vi "Read Attribute Data.vi"(8 "error in (no error)":errorcluster, 10 "Object Name":string, 11 "CS++Factory in":refnum<class "CS++Factory.lvclass">) -> (0 "error out":errorcluster, 2 "Attribute Data":variant, 3 "CS++Factory out":refnum<class "CS++Factory.lvclass">)   [LabVIEW 2013, in "CS++BaseClasses.lvlib" / "CS++Factory.lvclass"]
doc: "Read object attribute data from storage medium.\n\nThe default implementation reads from ini-file."
uses:
  CS++Factory.lvclass
  CS++Factory.lvclass/CS++Factory.ctl
  Libraries/Base/Error Definition.ctl
  <vilib>/Utility/config.llb/Read Key (String).vi
  <vilib>/Utility/config.llb/NI_LVConfig.lvlib
  Libraries/Base/CS++Base.lvlib
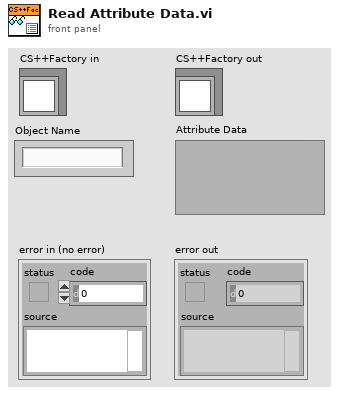
[diagram p1: front panel]
types:
  T1 = typedef "NI_LVConfig.lvlib/Config Data RefNum.ctl" = refnum<k1>
  T2 = typedef "CS++Base.lvlib/Error Definition.ctl" = u16
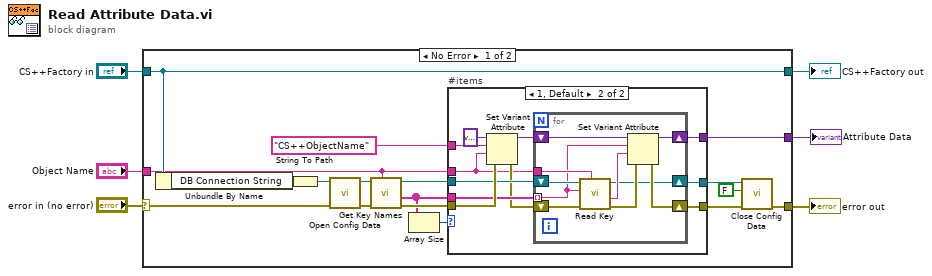
[diagram p0: block diagram]
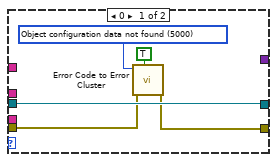
[diagram p2: hidden frame]
diagram:
  n1 = case shown="No Error" "error in (no error)" {
    selector: "error in (no error)" -> [w12 w51]
    tunnel: [w11 w51] -> w5
    tunnel: [w23 w50] -> w3
    tunnel: "CS++Factory in" -> [w23 w50]
    tunnel: [w10 _] -> w2
    tunnel: "Object Name" -> [w9 _]
    frame No Error {
      n2 = Unbundle By Name(w23) -> ("DB Connection String"=w22:string)
      n3 = String To Path(string=w22) -> (path=w13:path)
      n4 = call <vilib>:"Open Config Data.vi"("error in (no error)"=w12, "configuration file path"=w13) -> ("error out"=w16:errorcluster, "refnum"=w17:T1)  [unwired: 7 in, 1 out]
      n5 = call <vilib>:"Get Key Names.vi"("section"=w9, "error in (no error)"=w16, "refnum"=w17) -> ("error out"=w15:errorcluster, "key names"=w8:string[], "refnum out"=w14:T1)  [unwired: 5 in, 1 out]
      n6 = Array Size(array=w8) -> (size(s)=w7:i32)
      n7 = case "#items" shown="1, Default" w7 {
        tunnel: "CS++ObjectName" ("name") -> [_ w39]
        tunnel: [w28 w38] -> w20
        tunnel: [w26 w37] -> w19
        tunnel: w15 -> [w27 w36]
        tunnel: w14 -> [w28 w34]
        tunnel: w8 -> [_ w33]
        tunnel: [_ w30] -> w10
        tunnel: w9 -> [_ w29]
        frame 0 {
          w25 = T2 5000 items=["No Error"=0, "Object configuration data not found"=5000] ("CS++Error")
          n8 = call "Error Code to Error Cluster.vi"("show call chain? (False)"=TRUE, "Error In"=w27, "CS++Error"=w25) -> ("Error Out"=w26:errorcluster)  [unwired: 8 in]
        }
        frame 1, Default {
          n9 = Set Variant Attribute(Variant=variant ("variant"), name=w39, value=w29, error in=w36) -> (Variant out=w31:variant, error out=w32:errorcluster)  [unwired: 1 out]
          n10 = for {
            tunnel: w33 -> [w45] mode=indexing
            tunnel: w29 -> [w47]
            shift-right: [w42] -> w37
            shift-left: w32 -> [w48]
            shift-right: [w41] -> w30
            shift-left: w31 -> [w46]
            shift-right: [w40] -> w38
            shift-left: w34 -> [w49]
            n11 = call-poly <vilib>:"Read Key.vi"("section"=w47, "error in (no error)"=w48, "key"=w45, "refnum"=w49) -> ("error out"=w43:errorcluster, "value"=w44:string, "refnum out"=w40:T1)  [unwired: 4 in, 1 out]
            n12 = Set Variant Attribute(Variant=w46, name=w45, value=w44, error in=w43) -> (Variant out=w41:variant, error out=w42:errorcluster)  [unwired: 1 out]
          }
        }
      }
      n13 = call <vilib>:"Close Config Data.vi"("error in (no error)"=w19, "write file if changed (T)"=FALSE, "refnum"=w20) -> ("error out"=w11:errorcluster)  [unwired: 7 in, 1 out]
    }
    frame Error {
    }
  }
  "error out" <- w5
  "CS++Factory out" <- w3
  "Attribute Data" <- w2
